vi "Save_File_Dialog.vi"(8 "error in (no error)":errorcluster, 11 "Filename":string) -> (0 "error out":errorcluster, 2 "Cancelled":bool, 3 "Path":path)   [LabVIEW 2013]
doc: "Brings up a file dialog and, if necessary, a simple \"Overwrite file?\" dialog. Greatly decreases the likelihood of erros in file-related elements, especially in Query Dust Event."
uses:
  <userlib>/_OpenG.lib/file/file.llb/Strip Path Extension - Path__ogtk.vi
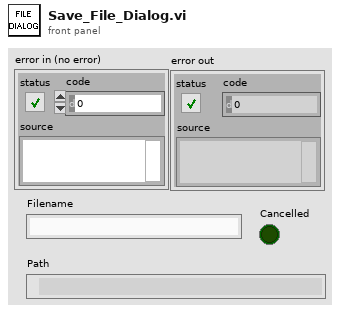
[diagram p1: front panel]
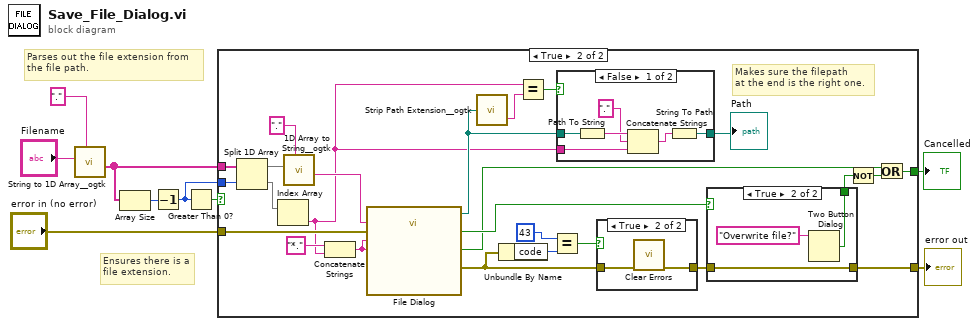
[diagram p0: block diagram]
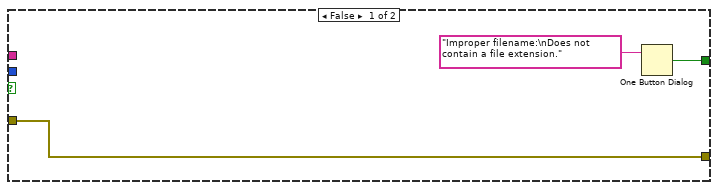
[diagram p2: hidden frame]
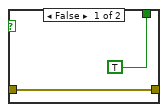
[diagram p5: hidden frame]
diagram:
  # "Parses out the file extension from\nthe file path."
  # "Ensures there is a\nfile extension."
  n1 = call <userlib>:"String to 1D Array__ogtk.vi"("delimiter (Tab)"=".", "string"="Filename") -> ("Array of Strings"=w3:string[])  [unwired: 9 in]
  n2 = Array Size(array=w3) -> (size(s)=w2:i32)
  n3 = Decrement(x=w2) -> (x-1=w1:i32)
  n4 = Greater Than 0?(x=w1) -> (x > 0?=w4:bool)
  n5 = case shown="True" w4 {
    tunnel: "error in (no error)" -> [w12 w30]
    tunnel: [w11 w29] -> w8
    tunnel: [w12 w28] -> w7
    tunnel: w3 -> [_ w27]
    tunnel: w1 -> [_ w26]
    frame False {
      n6 = One Button Dialog(message="Improper filename:\nDoes not contain a file extension.") -> (true=w11:bool)  [unwired: 1 in]
    }
    frame True {
      # "Makes sure the filepath\nat the end is the right one."
      n7 = Split 1D Array(array=w27, index=w26) -> (first subarray=w25:string[], second subarray=w23:string[])
      n8 = Index Array(array=w23) -> (element=w13:string)  [unwired: 1 in]
      n9 = call <userlib>:"1D Array to String__ogtk.vi"("delimiter (Tab)"=".", "Array of Strings"=w25) -> ("delimited string"=w17:string)  [unwired: 9 in]
      n10 = Concatenate Strings("*." ("string"), w13) -> (w21:string)
      n11 = call "File Dialog"("default name"=w17, "error in"=w30, "pattern (all files)"=w21, "pattern label"=w21) -> ("selected path"=w15:path, "exists"=w31:bool, "cancelled"=w20:bool, "error out"=w36:errorcluster)  [unwired: 8 in]
      n12 = call-poly <userlib>:"Strip Path Extension__ogtk.vi"("path"=w15) -> ("extension"=w18:string)  [unwired: 1 out]
      n13 = Unbundle By Name(w36) -> ("code"=w33:i32)
      n14 = Equal?(x=w13, y=w18) -> (x = y?=w16:bool)
      n15 = Equal?(x=43, y=w33) -> (x = y?=w35:bool)
      n16 = case shown="False" w16 {
        tunnel: w13 -> [w43 _]
        tunnel: w15 -> [w42 w44]
        tunnel: [w40 w44] -> w14
        frame False {
          n17 = Path To String(path=w42) -> (string=w39:string)
          n18 = Concatenate Strings(w39, "." ("string"), w43) -> (w41:string)
          n19 = String To Path(string=w41) -> (path=w40:path)
        }
        frame True {
        }
      }
      "Path" <- w14
      n20 = case shown="True" w35 {
        tunnel: w36 -> [w45 w47]
        tunnel: [w45 w46] -> w37
        frame False {
        }
        frame True {
          n21 = call <vilib>:"Clear Errors.vi"("error in (no error)"=w47) -> ("error out"=w46:errorcluster)  [unwired: 6 in]
        }
      }
      n22 = case shown="True" w31 {
        tunnel: [w49 w52] -> w28
        tunnel: w37 -> [w49 w52]
        tunnel: [TRUE ("T button?") w51] -> w32
        frame False {
        }
        frame True {
          n23 = Two Button Dialog(message="Overwrite file?") -> (T button?=w51:bool)  [unwired: 2 in]
        }
      }
      n24 = Not(x=w32) -> (.not. x?=w19:bool)
      n25 = Or(x=w20, y=w19) -> (x .or. y?=w29:bool)
    }
  }
  "error out" <- w7
  "Cancelled" <- w8
